vi "configuration UI.vi"() -> ()   [LabVIEW 2013, in "Profibus Module editor node.lvclass"]
uses:
  Profibus Module editor node.lvclass
  <vilib>/CEF_TreeControl/Node/NodeRef.ctl
  <vilib>/CEF_TreeControl/Node/NISE_CEF_Node.lvclass
  <vilib>/NI/AMC/Message Queue.ctl
  <vilib>/NI/AMC/Message.ctl
  <vilib>/NI/Tools/Keyed Array/KeyedArray.ctl
  <vilib>/CEF_TreeControl/Node/UserEventRef.ctl
  <vilib>/CEF_TreeControl/Controls/EventCluster.ctl
  <vilib>/NI/TBM Modules/Profibus/configuration/Profibus Module configuration.lvclass
  <vilib>/NI/Module Execution Interface/Engine Configuration/engine configuration.lvclass
  <vilib>/NI/Tag Bus Data Framework/Configuration Editor/Classes/Engine Parent/Engine Parent Editor Node.lvclass
  <vilib>/NI/Tag Bus/tag/tag descriptor.lvclass
  <vilib>/NI/Tag Bus/tag/Data Type.ctl
  <vilib>/NI/Tag Bus/tag/tag descriptor.lvclass/tag descriptor.ctl
  <vilib>/NI/Tag Bus Module Framework/root configuration/TBM configuration.lvclass/TBM configuration.ctl
  <vilib>/NI/Tag Bus/tag/write tag name.vi
  <vilib>/NI/Tag Bus/tag/write data type.vi
  <vilib>/NI/Tag Bus Module Framework/root configuration/Read instance name.vi
  <vilib>/NI/Tag Bus Data Framework/Configuration Editor/Classes/Module editor node/Read Module Configuration.vi
  <vilib>/NI/Tag Bus Module Framework/root configuration/create GUID.vi
  <vilib>/NI/Tag Bus Module Framework/root configuration/TBM configuration.lvclass
  <vilib>/NI/Tag Bus Module Framework/module configuration/TBM module configuration.lvclass
  <vilib>/CEF_TreeControl/NISE_CEF_TreeControl.lvlib
  <vilib>/NI/Tag Bus Data Framework/Configuration Editor/Classes/Module editor node/module editor node.lvclass
  <vilib>/NI/TBM Modules/Profibus/channel/Profibus channel.lvclass
  <vilib>/NI/Tools/Keyed Array/Tools_KeyedArray.lvlib
  <vilib>/NI/AMC/AMC.lvlib
panel:
  in  "Tab Control":enum32{"Static Configuration"}(tab)
  in  "Remove Button":bool
  in  "Add Button":bool
  in  "channel":i32(listbox)
  in  "settings":bool
  in  "user event":T1
  in  "main queue":T2
  in  "node ref":T3
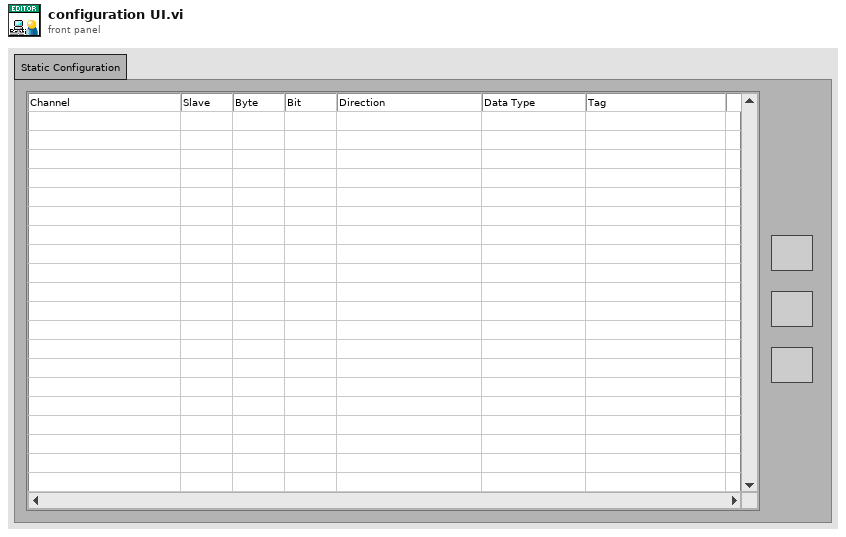
[diagram p1: front panel]
types:
  T1 = typedef "NISE_CEF_Node.lvclass/UserEventRef.ctl" = refnum<user-event>
  T2 = typedef "AMC.lvlib/Message Queue.ctl" = refnum<queue>
  T3 = typedef "NISE_CEF_Node.lvclass/NodeRef.ctl" = refnum<data-value>
  T4 = typedef "tag bus.lvlib/tag descriptor.lvclass/Data Type.ctl" = enum16{"Double", "Single", "I64", "I32", "I16", "I8", "U64", "U32", "U16", "U8", "Boolean", "String", "Array of Double", "Array of Single", "Array of I64", "Array of I32", "Array of I16", "Array of I8", "Array of U64", "Array of U32", "Array of U16", "Array of U8", "Array of Boolean", "Array of String"}
  T5 = typedef "NISE_CEF_TreeControl.lvlib/EventCluster.ctl" = cluster{"command":string, "data":string}
  T6 = typedef "Profibus Module editor node.lvclass/table line.ctl" = cluster{"profchan":refnum<class "Profibus channel.lvclass">, "tag name":string}
  T7 = typedef "LVPoint32TypeDef.ctl" = cluster{"Horizontal":i32, "Vertical":i32}
  T8 = typedef "LVRowAndColumnTypeDef.ctl" = cluster{"Row":i32, "Column":i32}
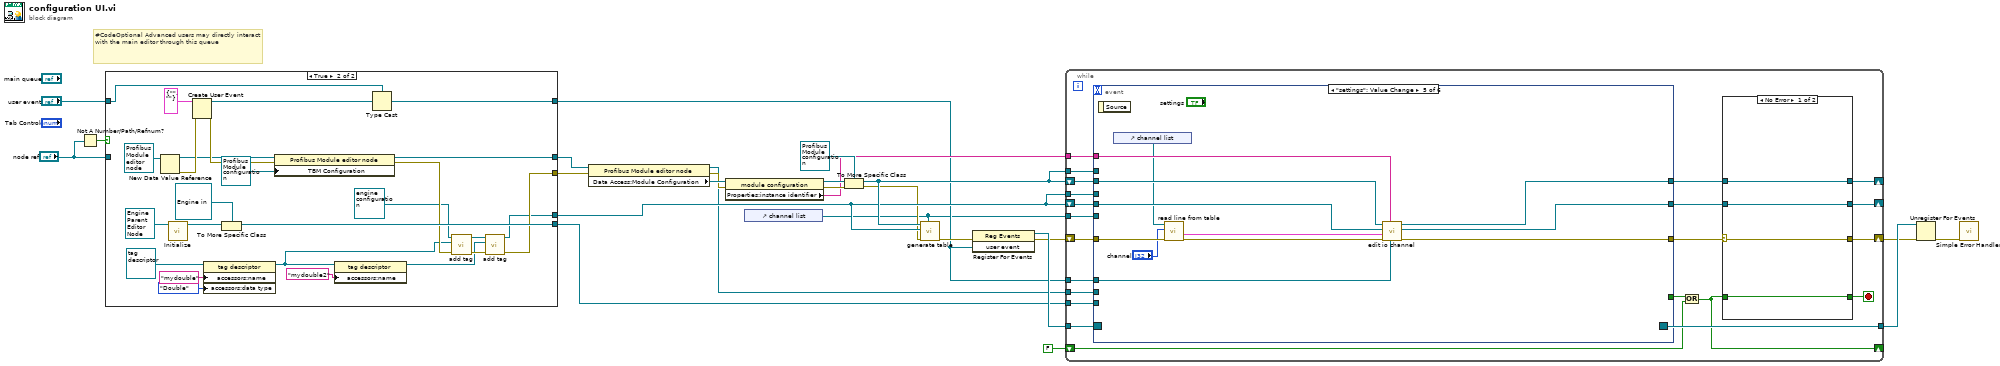
[diagram p0: block diagram]
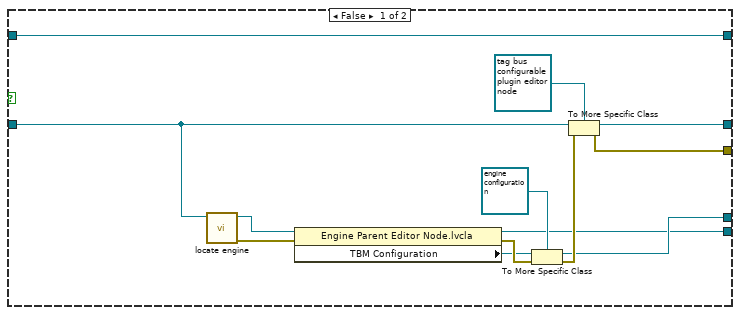
[diagram p2: hidden frame]
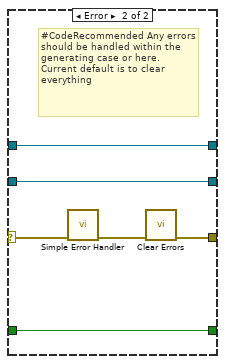
[diagram p3: hidden frame]
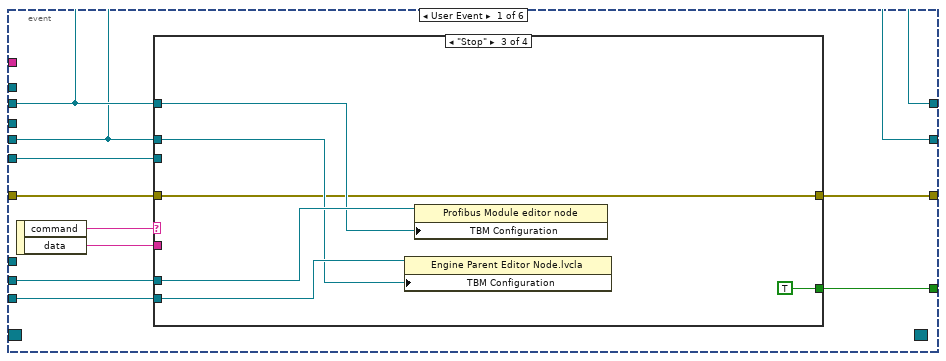
[diagram p4: hidden frame]
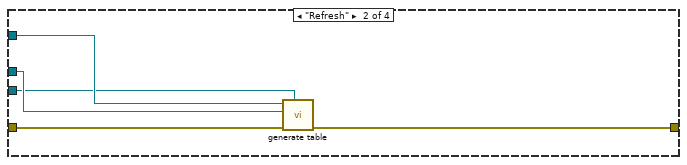
[diagram p6: hidden frame]
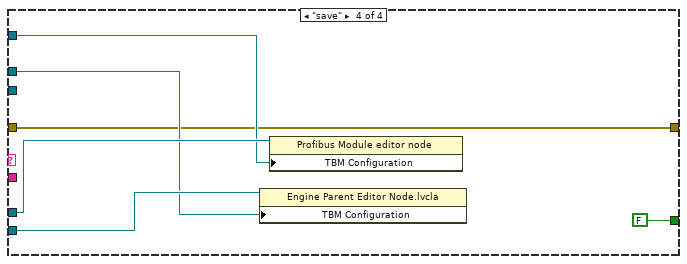
[diagram p7: hidden frame]
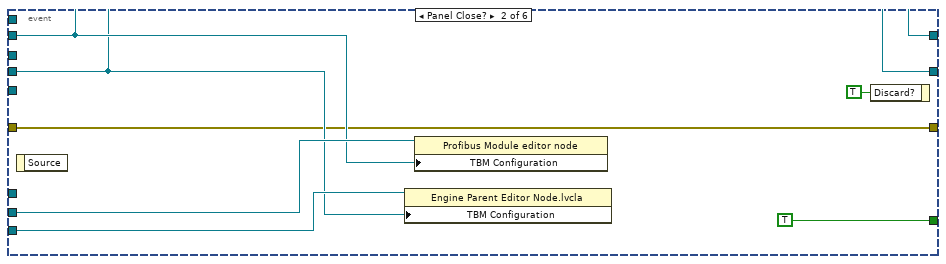
[diagram p8: hidden frame]
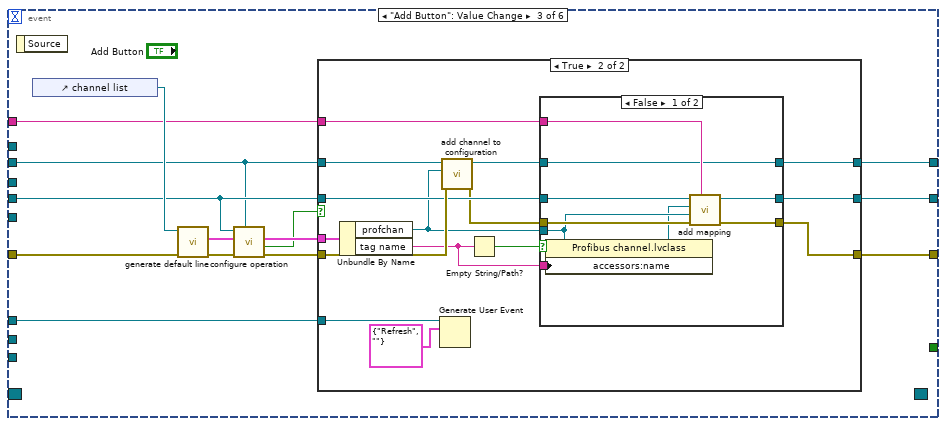
[diagram p9: hidden frame]
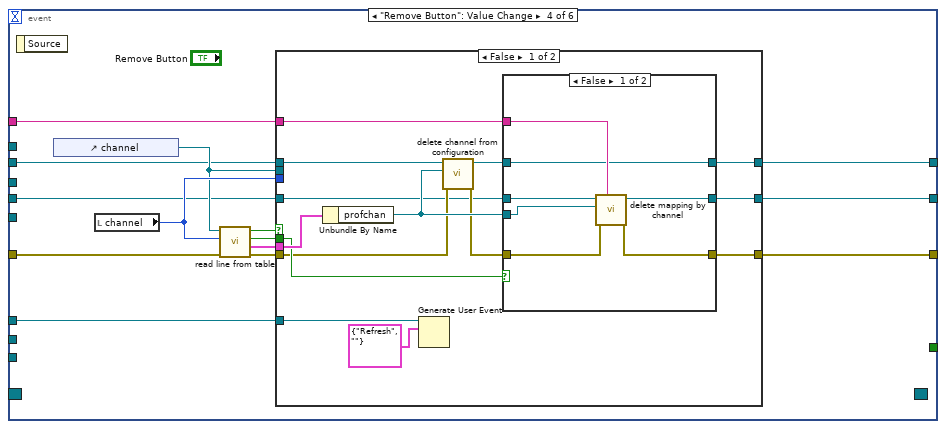
[diagram p12: hidden frame]
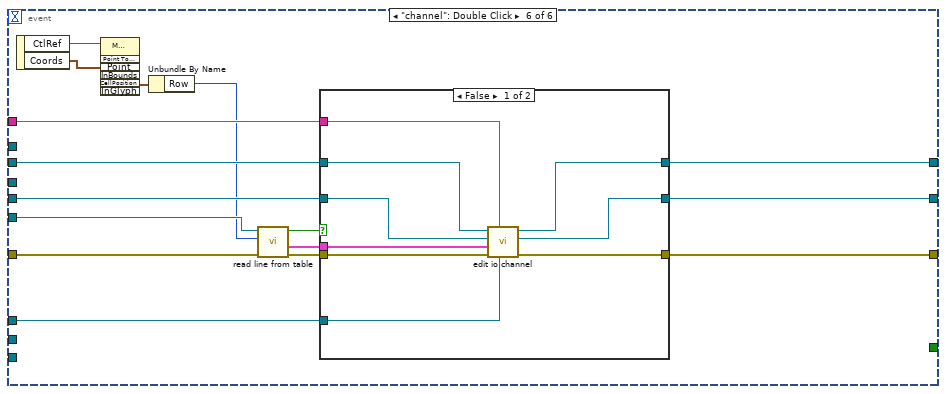
[diagram p15: hidden frame]
diagram:
  # "#CodeOptional Advanced users may directly interact with the main editor through this queue"
  n1 = Not A Number/Path/Refnum?(number/path/refnum="node ref") -> (NaN/Path/Refnum?=w16:bool)
  n2 = case shown="True" w16 {
    tunnel: "user event" -> [w38 w40]
    tunnel: [w38 w41] -> w2
    tunnel: "node ref" -> [w36 _]
    tunnel: [w35 w58] -> w8
    tunnel: [w34 w45] -> w14
    tunnel: [w27 w44] -> w10
    tunnel: [w26 w55] -> w4
    frame False {
      n3 = call <vilib>:"locate engine.vi"("component"=w36) -> ("error out"=w31:errorcluster, "engine"=w33:refnum<data-value>)  [unwired: 9 in]
      n4 = property class="Engine Parent Editor Node.lvcla"(reference=w33, error in=w31) -> (reference out=w26:refnum<data-value>, error out=w30:errorcluster, "TBM Configuration"=w29:refnum<class "TBM configuration.lvclass">)
      n5 = To More Specific Class(target class=refnum<class "engine configuration.lvclass"> refnum ("engine configuration.lvclass"), reference=w29, error in=w30) -> (specific class reference=w27:refnum<class "engine configuration.lvclass">, error out=w28:errorcluster)
      n6 = To More Specific Class(target class=refnum<data-value> refnum ("data value reference"), reference=w36, error in=w28) -> (specific class reference=w35:refnum<data-value>, error out=w34:errorcluster)
    }
    frame True {
      n7 = New Data Value Reference(data value=refnum<class "Profibus Module editor node.lvclass"> refnum ("tag bus configurable plugin editor node")) -> (data value reference=w57:refnum<data-value>, error out=w60:errorcluster)  [unwired: 1 in]
      n8 = call-dynamic "Initialize.vi"("Engine in"=refnum<class "Engine Parent Editor Node.lvclass"> refnum) -> ("data value reference"=w56:T3)  [unwired: 8 in, 2 out]
      n9 = Create User Event(user event datatype=T5 {"command"="", "data"=""} ("event data"), error in=w60) -> (user event=w63:refnum<user-event>, error out=w59:errorcluster)
      n10 = property class="tag descriptor"(reference=refnum<class "tag descriptor.lvclass"> refnum ("tag descriptor"), "accessors:name"="mydouble" ("name"), "accessors:data type"=Data_Type."Double" ("data type")) -> (reference out=w42:refnum<class "tag descriptor.lvclass">)  [unwired: 1 in, 1 out]
      n11 = To More Specific Class(target class=refnum<data-value> refnum ("data value reference"), reference=w56) -> (specific class reference=w55:refnum<data-value>)  [unwired: 1 in, 1 out]
      n12 = property class="Profibus Module editor node"(reference=w57, error in=w59, "TBM Configuration"=refnum<class "Profibus Module configuration.lvclass"> refnum ("tag bus configurable plugin module configuration")) -> (reference out=w58:refnum<data-value>, error out=w49:errorcluster)
      n13 = property class="tag descriptor"(reference=w42, "accessors:name"="mydouble2" ("name")) -> (reference out=w43:refnum<class "tag descriptor.lvclass">)  [unwired: 1 in, 1 out]
      n14 = Type Cast(type=w40, x=w63) -> (*(type *) &x=w41:T1)
      n15 = call <vilib>:"add tag.vi"("error in"=w49, "tag descriptor"=w42, "engine configuration in"=refnum<class "engine configuration.lvclass"> refnum ("Engine Configuration")) -> ("error out"=w47:errorcluster, "engine configuration out"=w46:refnum<class "engine configuration.lvclass">)  [unwired: 7 in]
      n16 = call <vilib>:"add tag.vi"("error in"=w47, "tag descriptor"=w43, "engine configuration in"=w46) -> ("error out"=w45:errorcluster, "engine configuration out"=w44:refnum<class "engine configuration.lvclass">)  [unwired: 7 in]
    }
  }
  n17 = property class="Profibus Module editor node"(reference=w8, error in=w14) -> (reference out=w5:refnum<data-value>, error out=w19:errorcluster, "Data Access:Module Configuration"=w20:refnum<class "TBM module configuration.lvclass">)
  n18 = property class="module configuration"(reference=w20, error in=w19) -> (reference out=w17:refnum<class "TBM module configuration.lvclass">, error out=w18:errorcluster, "Properties:instance identifier"=w13:string)
  n19 = control-ref of="channel list"() -> (w1:refnum<vi>)
  n20 = To More Specific Class(target class=refnum<class "Profibus Module configuration.lvclass"> refnum ("tag bus configurable plugin module configuration"), reference=w17, error in=w18) -> (specific class reference=w11:refnum<class "Profibus Module configuration.lvclass">, error out=w9:errorcluster)
  n21 = call "generate table.vi"("table"=w1, "error in"=w9, "engine configuration in"=w10, "Profibus Module configuration in"=w11) -> ("error out"=w7:errorcluster)  [unwired: 7 in]
  n22 = register-events(error in=w7, w2) -> (reference out=w25:refnum<event-registration>, error out=w6:errorcluster)  [unwired: 1 in]
  n23 = while {
    tunnel: w25 -> [w86]
    tunnel: [w85] -> w24
    shift-right: [w79] -> w23
    shift-left: w6 -> [w84]
    shift-right: [w81] -> _
    shift-left: FALSE -> [w80]
    tunnel: w11 -> [w77]
    shift-right: [w73] -> _
    shift-left: w11 -> [w78]
    shift-right: [w74] -> _
    shift-left: w10 -> [w75]
    tunnel: w10 -> [w76]
    tunnel: w13 -> [w72]
    tunnel: w5 -> [w69]
    tunnel: w4 -> [w68]
    tunnel: w2 -> [w67]
    tunnel: w1 -> [w65]
    stop <- w83 stop-if-true
    n24 = event shown="[4] \"settings\": Value Change" {
      selector: w86 -> [_ _ _ _ _ _]
      dyn-events: [_ _ _ _ _ _] -> w85
      timeout: _ -> [_ _ _ _ _ _]
      tunnel: [w106 TRUE _ _ _ _] -> w82
      tunnel: [w98 w126 w145 w189 w219 w243] -> w66
      tunnel: w84 -> [w99 w126 w144 w188 w228 w244]
      tunnel: w78 -> [w102 w128 w132 w184 w224 w239]
      tunnel: w77 -> [_ _ _ _ _ _]
      tunnel: w76 -> [_ _ _ _ _ _]
      tunnel: w75 -> [w101 w127 w134 w183 w225 w240]
      tunnel: [w101 w127 w138 w178 w222 w237] -> w71
      tunnel: [w102 w128 w137 w177 w223 w238] -> w70
      tunnel: w72 -> [_ _ w133 w179 w221 w236]
      tunnel: w69 -> [w104 w130 _ _ _ _]
      tunnel: w68 -> [w103 w129 _ _ _ _]
      tunnel: w67 -> [_ _ w135 w176 w220 w235]
      tunnel: w65 -> [w97 _ _ _ _ w234]
      event User Event {
        n25 = event-data() -> ("command"=w105:string, "data"=w100:string)  [unwired: 1 in]
        n26 = case shown="\"Stop\"" w105 {
          tunnel: [_ _ TRUE FALSE] -> w106
          tunnel: w104 -> [_ _ w117 w123]
          tunnel: w103 -> [_ _ w116 w122]
          tunnel: w102 -> [_ w112 w115 w121]
          tunnel: w101 -> [_ w111 w114 w120]
          tunnel: w100 -> [_ _ _ _]
          tunnel: w99 -> [w107 w110 w113 w119]
          tunnel: [w107 w109 w113 w119] -> w98
          tunnel: w97 -> [_ w108 _ _]
          frame Default {
          }
          frame "Refresh" {
            n27 = call "generate table.vi"("table"=w108, "error in"=w110, "engine configuration in"=w111, "Profibus Module configuration in"=w112) -> ("error out"=w109:errorcluster)  [unwired: 7 in]
          }
          frame "Stop" {
            n28 = property class="Engine Parent Editor Node.lvcla"(reference=w116, "TBM Configuration"=w114) -> ()  [unwired: 1 in, 2 out]
            n29 = property class="Profibus Module editor node"(reference=w117, "TBM Configuration"=w115) -> ()  [unwired: 1 in, 2 out]
          }
          frame "save" {
            n30 = property class="Engine Parent Editor Node.lvcla"(reference=w122, "TBM Configuration"=w120) -> ()  [unwired: 1 in, 2 out]
            n31 = property class="Profibus Module editor node"(reference=w123, "TBM Configuration"=w121) -> ()  [unwired: 1 in, 2 out]
          }
        }
      }
      event Panel Close? {
        n32 = event-data() -> ()  [unwired: 1 in, 1 out]
        n33 = property class="Engine Parent Editor Node.lvcla"(reference=w129, "TBM Configuration"=w127) -> ()  [unwired: 1 in, 2 out]
        n34 = property class="Profibus Module editor node"(reference=w130, "TBM Configuration"=w128) -> ()  [unwired: 1 in, 2 out]
        n35 = event-data("Discard?"=TRUE) -> ()  [unwired: 1 in, 1 out]
      }
      event "Add Button": Value Change {
        n36 = event-data() -> ()  [unwired: 1 in, 1 out]
        n37 = control-ref of="channel list"() -> (w143:refnum<vi>)
        n38 = call "generate default line.vi"("error in"=w144, "operations table"=w143) -> ("error out"=w141:errorcluster, "line"=w142:T6)  [unwired: 8 in]
        n39 = call "configure operation.vi"("owner ID"=w132, "error in"=w141, "line item in"=w142, "engine configuration in"=w134) -> ("error out"=w139:errorcluster, "success"=w136:bool, "line item out"=w140:T6)  [unwired: 4 in, 1 out]
        n40 = case shown="True" w136 {
          tunnel: [w148 w151] -> w145
          tunnel: w139 -> [w148 w161]
          tunnel: w134 -> [w147 w159]
          tunnel: w140 -> [_ w162]
          tunnel: w132 -> [w146 w163]
          tunnel: [w147 w158] -> w138
          tunnel: [w146 w152] -> w137
          tunnel: w133 -> [_ w155]
          tunnel: w135 -> [_ w150]
          frame False {
          }
          frame True {
            n41 = Unbundle By Name(w162) -> ("profchan"=w156:refnum<class "Profibus channel.lvclass">, "tag name"=w154:string)
            n42 = Generate User Event(user event=w150, event data cluster=T5 {"command"="Refresh", "data"=""} ("event data")) -> ()  [unwired: 2 in, 2 out]
            n43 = call <vilib>:"add channel to configuration.vi"("error in"=w161, "TBM channel in"=w156, "Profibus Module configuration in"=w163) -> ("error out"=w157:errorcluster, "Profibus Module configuration out"=w153:refnum<class "Profibus Module configuration.lvclass">)  [unwired: 7 in]
            n44 = Empty String/Path?(string/path=w154) -> (empty?=w160:bool)
            n45 = case shown="False" w160 {
              tunnel: w159 -> [w172 w175]
              tunnel: [w171 w175] -> w158
              tunnel: w157 -> [w170 w174]
              tunnel: w156 -> [w168 _]
              tunnel: w155 -> [w169 _]
              tunnel: w154 -> [w167 _]
              tunnel: [w165 w174] -> w151
              tunnel: w153 -> [w164 w173]
              tunnel: [w164 w173] -> w152
              frame False {
                n46 = property class="Profibus channel.lvclass"(reference=w168, "accessors:name"=w167) -> (reference out=w166:refnum<class "Profibus channel.lvclass">)  [unwired: 1 in, 1 out]
                n47 = call <vilib>:"add mapping.vi"("owner ID"=w169, "error in"=w170, "channel"=w168, "tag descriptor"=w166, "engine configuration"=w172) -> ("error out"=w165:errorcluster, "engine configuration out"=w171:refnum<class "engine configuration.lvclass">)  [unwired: 5 in]
              }
              frame True {
              }
            }
          }
        }
      }
      event "Remove Button": Value Change {
        n48 = event-data() -> ()  [unwired: 1 in, 1 out]
        n49 = control-ref of="channel"() -> (w186:refnum<vi>)
        n50 = local read "channel"() -> (w187:i32)
        n51 = call "read line from table.vi"("error in"=w188, "line number"=w187, "channels table"=w186) -> ("error out"=w180:errorcluster, "line"=w185:T6, "empty tag?"=w181:bool, "empty channel?"=w182:bool)  [unwired: 5 in]
        n52 = case shown="False" w182 {
          tunnel: [w192 w215] -> w189
          tunnel: w187 -> [_ _]
          tunnel: w186 -> [_ _]
          tunnel: w185 -> [w203 _]
          tunnel: w184 -> [w201 w214]
          tunnel: w183 -> [w196 w216]
          tunnel: w181 -> [w202 _]
          tunnel: w180 -> [w199 w215]
          tunnel: w179 -> [w195 _]
          tunnel: [w194 w216] -> w178
          tunnel: [w193 w214] -> w177
          tunnel: w176 -> [w190 _]
          frame False {
            n53 = Unbundle By Name(w203) -> ("profchan"=w200:refnum<class "Profibus channel.lvclass">)
            n54 = Generate User Event(user event=w190, event data cluster=T5 {"command"="Refresh", "data"=""} ("event data")) -> ()  [unwired: 2 in, 2 out]
            n55 = call <vilib>:"delete channel from configuration.vi"("error in"=w199, "TBM channel in"=w200, "Profibus Module configuration in"=w201) -> ("error out"=w197:errorcluster, "Profibus Module configuration out"=w198:refnum<class "Profibus Module configuration.lvclass">)  [unwired: 7 in]
            n56 = case shown="False" w202 {
              tunnel: w200 -> [w209 _]
              tunnel: w198 -> [w204 w211]
              tunnel: w197 -> [w207 w212]
              tunnel: w196 -> [w210 w213]
              tunnel: w195 -> [w208 _]
              tunnel: [w206 w213] -> w194
              tunnel: [w205 w212] -> w192
              tunnel: [w204 w211] -> w193
              frame False {
                n57 = call <vilib>:"delete mapping by channel.vi"("owner ID"=w208, "error in"=w207, "channel"=w209, "engine configuration in"=w210) -> ("error out"=w205:errorcluster, "engine configuration out"=w206:refnum<class "engine configuration.lvclass">)  [unwired: 6 in]
              }
              frame True {
              }
            }
          }
          frame True {
          }
        }
      }
      event "settings": Value Change {
        n58 = event-data() -> ()  [unwired: 1 in, 1 out]
        n59 = control-ref of="channel list"() -> (w217:refnum<vi>)
        n60 = call "read line from table.vi"("error in"=w228, "line number"="channel", "channels table"=w217) -> ("error out"=w227:errorcluster, "line"=w226:T6)  [unwired: 5 in, 2 out]
        n61 = call "edit io channel.vi"("user event"=w220, "instance identifier"=w221, "error in"=w227, "line"=w226, "engine configuration in"=w225, "Profibus Module configuration in"=w224) -> ("error out"=w219:errorcluster, "engine configuration out"=w222:refnum<class "engine configuration.lvclass">, "Profibus Module configuration out"=w223:refnum<class "Profibus Module configuration.lvclass">)  [unwired: 3 in]
      }
      event "channel": Double Click {
        n62 = event-data() -> ("CtlRef"=w233:refnum<vi>, "Coords"=w232:T7)  [unwired: 1 in]
        n63 = invoke class="MCListbox (strict)" method="Point To Row Column"(reference=w233, "Point"=w232) -> ("CellPosition"=w231:T8)  [unwired: 5 in, 6 out]
        n64 = Unbundle By Name(w231) -> ("Row"=w230:i32)
        n65 = call "read line from table.vi"("error in"=w244, "line number"=w230, "channels table"=w234) -> ("error out"=w242:errorcluster, "line"=w241:T6, "empty channel?"=w229:bool)  [unwired: 5 in, 1 out]
        n66 = case shown="False" w229 {
          tunnel: [w253 w254] -> w243
          tunnel: w242 -> [w252 w254]
          tunnel: w241 -> [w251 _]
          tunnel: w240 -> [w250 w255]
          tunnel: w239 -> [w249 w256]
          tunnel: [w248 w256] -> w238
          tunnel: [w247 w255] -> w237
          tunnel: w236 -> [w246 _]
          tunnel: w235 -> [w245 _]
          frame False {
            n67 = call "edit io channel.vi"("user event"=w245, "instance identifier"=w246, "error in"=w252, "line"=w251, "engine configuration in"=w250, "Profibus Module configuration in"=w249) -> ("error out"=w253:errorcluster, "engine configuration out"=w247:refnum<class "engine configuration.lvclass">, "Profibus Module configuration out"=w248:refnum<class "Profibus Module configuration.lvclass">)  [unwired: 3 in]
          }
          frame True {
          }
        }
      }
    }
    n68 = Or(x=w82, y=w80) -> (x .or. y?=w81:bool)
    n69 = case shown="No Error" w66 {
      selector: w66 -> [w87 w95]
      tunnel: [w90 w96] -> w83
      tunnel: w81 -> [w90 w96]
      tunnel: [w87 w93] -> w79
      tunnel: w71 -> [w88 w92]
      tunnel: [w88 w92] -> w74
      tunnel: w70 -> [w89 w91]
      tunnel: [w89 w91] -> w73
      frame No Error {
      }
      frame Error {
        # "#CodeRecommended Any errors should be handled within the generating case or here. Current default is to clear everything"
        n70 = call <vilib>:"Simple Error Handler.vi"("error in (no error)"=w95) -> ("error out"=w94:errorcluster)  [unwired: 4 in, 4 out]
        n71 = call <vilib>:"Clear Errors.vi"("error in (no error)"=w94) -> ("error out"=w93:errorcluster)  [unwired: 6 in]
      }
    }
  }
  n72 = Unregister For Events(event registration refnum=w24, error in=w23) -> (error out=w3:errorcluster)
  n73 = call <vilib>:"Simple Error Handler.vi"("error in (no error)"=w3) -> ()  [unwired: 4 in, 5 out]
